vi "FindAndInitializeNextron.vi"(8 "error in (no error)":errorcluster) -> (0 "error in (no error) 2":errorcluster, 3 "VISA Refnum Out":refnum<visa-resource-name>)   [LabVIEW 2023]
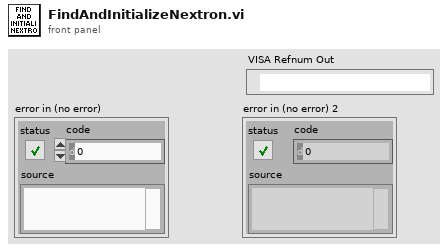
[diagram p1: front panel]
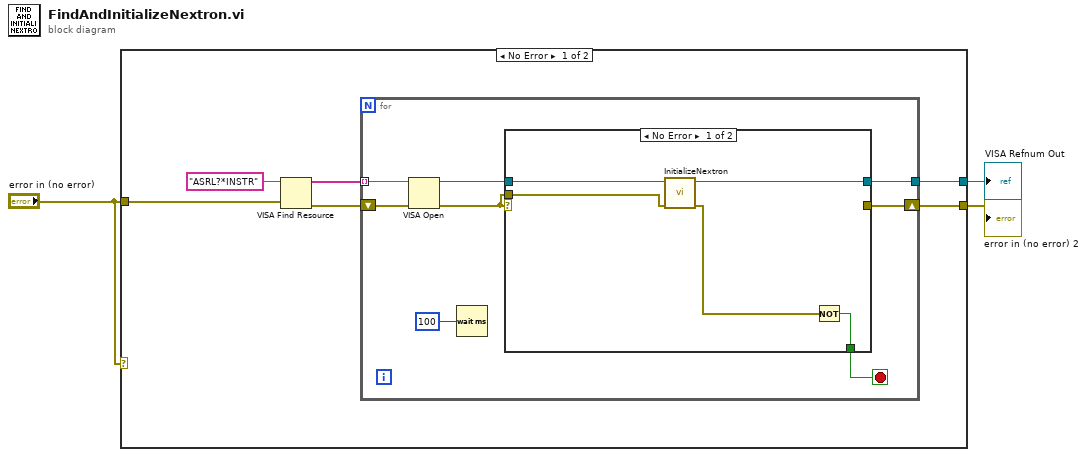
[diagram p0: block diagram]
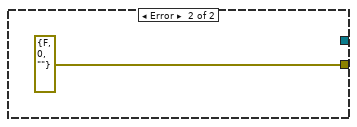
[diagram p2: hidden frame]
diagram:
  n1 = case shown="No Error" "error in (no error)" {
    tunnel: "error in (no error)" -> [w7 w24]
    tunnel: [w6 _] -> w2
    tunnel: [w5 w24] -> w1
    frame No Error {
      n2 = VISA Find Resource(8:w7, 11:"ASRL?*INSTR" ("expression (\"?*\")")) -> (0:w4:errorcluster, 3:w8:string[])  [unwired: 1 in, 1 out]
      n3 = for {
        tunnel: w8 -> [w17] mode=indexing
        shift-right: [w14] -> w5
        shift-left: w4 -> [w16]
        tunnel: [w12] -> w6
        stop <- w11 stop-if-true
        n4 = VISA Open(error in (no error)=w16, VISA resource name=w17) -> (VISA resource name=w15:refnum<visa-resource-name>, error out=w13:errorcluster)  [unwired: 3 in]
        n5 = Wait (ms)(milliseconds to wait=u32 100) -> ()  [unwired: 1 out]
        n6 = case shown="No Error" w13 {
          tunnel: w15 -> [w22 _]
          tunnel: [_ errorcluster {"status"=FALSE, "code"=0, "source"=""} ("error constant")] -> w14
          tunnel: w13 -> [w21 _]
          tunnel: [w20 _] -> w12
          tunnel: [w19 _] -> w11
          frame No Error {
            n7 = call "InitializeNextron.vi"("error in (no error)"=w21, "VISA Refnum in"=w22) -> ("error in (no error) 2"=w18:errorcluster, "VISA Refnum Out"=w20:refnum<visa-resource-name>)  [unwired: 7 in, 1 out]
            n8 = Not(x=w18) -> (.not. x?=w19:bool)
          }
          frame Error {
          }
        }
      }
    }
    frame Error {
    }
  }
  "VISA Refnum Out" <- w2
  "error in (no error) 2" <- w1
